vi "Read table servicios.vi"(8 "error in (no error)":errorcluster, 11 "Contabilidad in":refnum<class "Contabilidad.lvclass">) -> (0 "error out":errorcluster, 3 "Contabilidad out":refnum<class "Contabilidad.lvclass">)   [LabVIEW 2020, in "Contabilidad.lvlib" / "Contabilidad.lvclass"]
uses:
  Contabilidad.lvclass
  Contabilidad.lvclass/Contabilidad.ctl
  <vilib>/drjdpowell/SQLite Library/SQL Connection/Open (path).vi
  <vilib>/drjdpowell/SQLite Library/SQL Connection/Open (string).vi
  <vilib>/AdvancedString/Path To Command Line String.vi
  <vilib>/drjdpowell/SQLite Library/SQL Connection/Execute SQL.vi
  <vilib>/drjdpowell/SQLite Library/SQL Connection/Connection.lvclass
  <vilib>/drjdpowell/SQLite Library/SQLite.lvlib
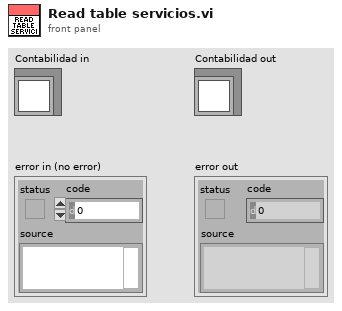
[diagram p1: front panel]
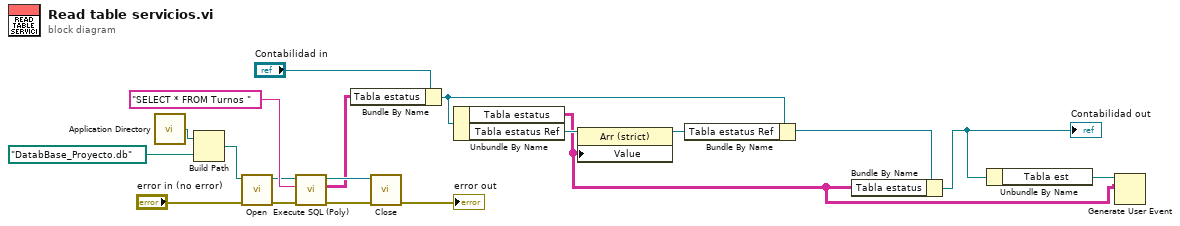
[diagram p0: block diagram]
diagram:
  n1 = call <vilib>:"Application Directory.vi"() -> ("Application Directory"=w16:path)
  n2 = Build Path(base path=w16, name or relative path=path "DatabBase_Proyecto.db") -> (appended path=w14:path)
  n3 = call-poly <vilib>:"Open.vi"("error in (no error)"="error in (no error)", "db file"=w14) -> ("error out"=w18:errorcluster, "SQLite Connection"=w13:refnum<class "Connection.lvclass">)  [unwired: 8 in]
  n4 = call-poly <vilib>:"Execute SQL (Poly).vi"("error in (no error)"=w18, "SQL"="SELECT * FROM Turnos ", "SQLite Connection in"=w13) -> ("error out"=w19:errorcluster, "Result Set"=w8:string[][], "SQLite Connection"=w12:refnum<class "Connection.lvclass">)  [unwired: 5 in, 1 out]
  n5 = Bundle By Name(cluster="Contabilidad in", "Tabla estatus"=w8) -> (w7:refnum<class "Contabilidad.lvclass">)
  n6 = call-dynamic "Close.vi"("error in (no error)"=w19, "SQLite Connection in"=w12) -> ("error out"=→"error out":errorcluster)  [unwired: 9 in]
  n7 = Unbundle By Name(w7) -> ("Tabla estatus"=w1:string[][], "Tabla estatus Ref"=w6:refnum<vi>)
  n8 = property class="Arr (strict)"(reference=w6, "Value"=w1) -> (reference out=w5:refnum<vi>)  [unwired: 1 in, 1 out]
  n9 = Bundle By Name(cluster=w7, "Tabla estatus Ref"=w5) -> (w4:refnum<class "Contabilidad.lvclass">)
  n10 = Bundle By Name(cluster=w4, "Tabla estatus"=w1) -> (w3:refnum<class "Contabilidad.lvclass">)
  "Contabilidad out" <- w3
  n11 = Unbundle By Name(w3) -> ("Tabla est"=w2:refnum<user-event>)
  n12 = Generate User Event(user event=w2, event data cluster=w1) -> ()  [unwired: 2 in, 2 out]
